vi "Pre-Request.vi"(6 "timeout":i32, 8 "error in (no error)":errorcluster, 9 "url":string, 10 "request-specific headers":T1[](array[typedef]), 11 "REST Client in":refnum<class "REST Client.lvclass">) -> (0 "error out":errorcluster, 1 "Resolved URL":string, 2 "http-client":refnum<class "http-client.lvclass">, 3 "REST Client out":refnum<class "REST Client.lvclass">, 4 "Timeout":i32)   [LabVIEW 2020, in "REST Client.lvlib" / "REST Client.lvclass"]
uses:
  REST Client.lvclass
  http-client/http-client.lvclass
  HTTP Header.ctl
  REST Client.lvclass/REST Client.ctl
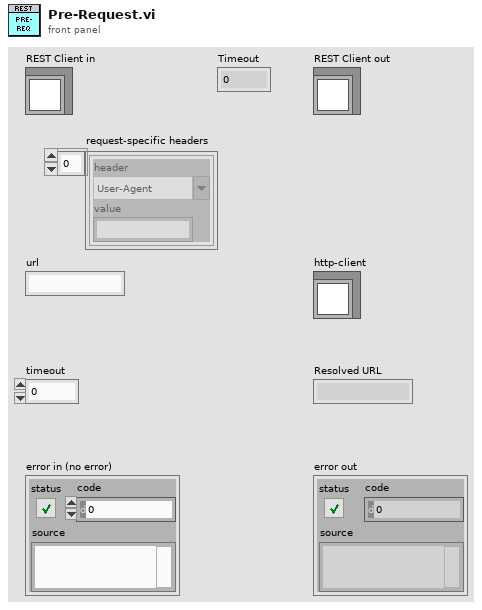
[diagram p1: front panel]
types:
  T1 = typedef "REST Client.lvlib/REST Client.lvclass/HTTP Header.ctl" = cluster{"header":string, "value":string}
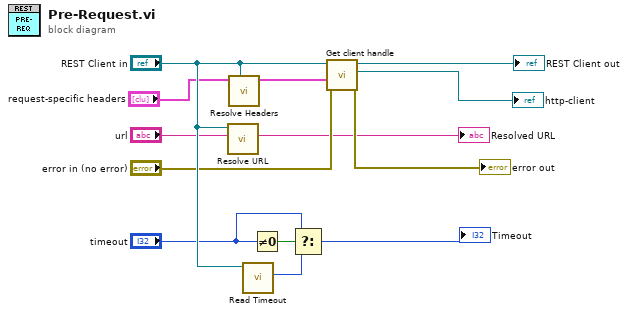
[diagram p0: block diagram]
diagram:
  n1 = call "Resolve URL.vi"("Path"="url", "REST Client in"="REST Client in") -> ("Resolved URL"=→"Resolved URL":string)  [unwired: 9 in]
  n2 = call "Resolve Headers.vi"("REST Client in"="REST Client in", "headers in"="request-specific headers") -> ("headers out"=w12:T1[])  [unwired: 9 in]
  n3 = call-dynamic "Read Timeout.vi"("REST Client in"="REST Client in") -> ("Timeout"=w9:i32)  [unwired: 8 in, 2 out]
  n4 = Not Equal To 0?(x="timeout") -> (x != 0?=w5:bool)
  n5 = Select(t="timeout", s=w5, f=w9) -> (s? t:f=→"Timeout":i32)
  n6 = call "Get client handle.vi"("error in (no error)"="error in (no error)", "headers"=w12, "REST Client in"="REST Client in") -> ("error out"=→"error out":errorcluster, "http-client"=→"http-client":refnum<class "http-client.lvclass">, "REST Client out"=→"REST Client out":refnum<class "REST Client.lvclass">)  [unwired: 6 in]
